vi "InnerCallbackOnLoadUI.vi"(8 "error in":errorcluster, 10 "node (for type)":refnum<class "NISE_CEF_Node.lvclass">, 11 "node reference":refnum<data-value>) -> (0 "error out":errorcluster)   [LabVIEW 2013, in "NISE_CEF_Node.lvclass"]
uses:
  NISE_CEF_Node.lvclass
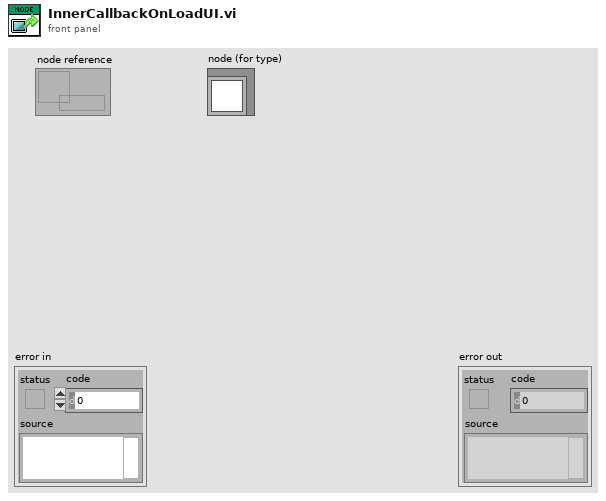
[diagram p1: front panel]
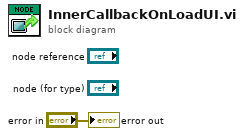
[diagram p0: block diagram]
diagram:
  "error out" <- "error in"
